vi "tearDown.vi"(8 "error in (no error)":errorcluster, 11 "reference in":refnum<class "FPGA Addon Test Class.lvclass">) -> (0 "error out":errorcluster, 3 "reference out":refnum<class "FPGA Addon Test Class.lvclass">)   [LabVIEW 2019]
doc: "tearDown runs after the test method has completed. Use this method to clean up any operations or references that were opened by setUp or the test method. Unit tests should be independent of other unit tests so this VI should ensure that the next test can run in a 'clean' test environment."
uses:
  FPGA Addon Test Class.lvclass
  C:/Program Files (x86)/National Instruments/LabVIEW 2019/vi.lib/NI/NI VeriStand Development Tools/NI Veristand Test Utilities/VeriStandTestCase/VeriStandTestCase.lvclass
  C:/Program Files (x86)/National Instruments/LabVIEW 2019/vi.lib/addons/_JKI Toolkits/VI Tester/TestCase.llb/TestCase.lvclass
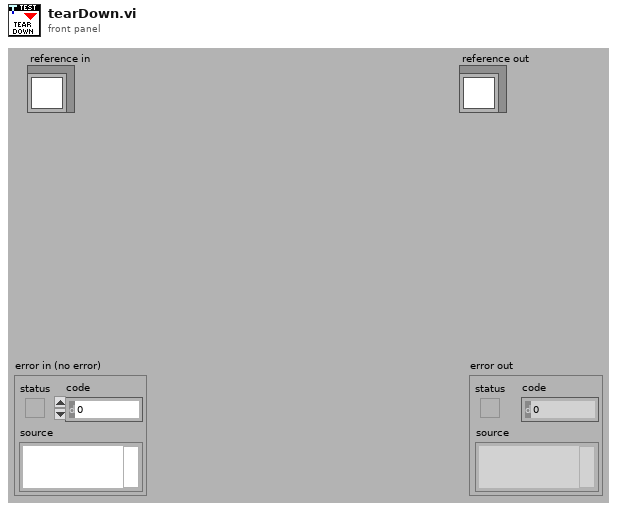
[diagram p1: front panel]
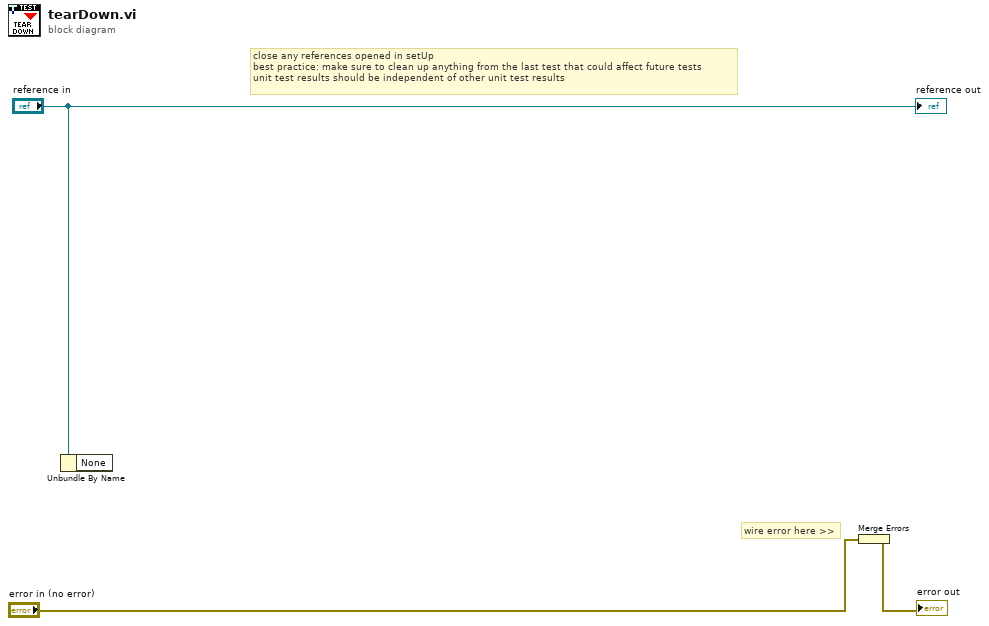
[diagram p0: block diagram]
diagram:
  # "wire error here >>"
  # "close any references opened in setUp\nbest practice: make sure to clean up anything from the last test that could affect future tests\nunit test results should be independent of other unit test results"
  n1 = Unbundle By Name("reference in") -> ()  [unwired: 1 out]
  n2 = Merge Errors("error in (no error)") -> (→"error out":errorcluster)
  "reference out" <- "reference in"
